vi "Control Car.vi"(8 "error in (no error)":errorcluster, 9 "Throttle":sgl, 10 "Steering":sgl, 11 "FormulaG API in":refnum<class "FormulaG API.lvclass">) -> (0 "error out":errorcluster, 3 "FormulaG API out":refnum<class "FormulaG API.lvclass">)   [LabVIEW 2020, in "FormulaG.lvlib" / "FormulaG API.lvclass"]
uses:
  FormulaG API.lvclass
  FormulaLV-Common/Car Control.ctl
  Command.ctl
  FormulaG API.lvclass/FormulaG API.ctl
  <vilib>/IlluminatedG/lv-stream/stream/Stream.lvclass/Stream.ctl
  <vilib>/IlluminatedG/lv-stream/stream/Dispatch Sniffer Data.vi
  <vilib>/IlluminatedG/lv-stream/stream/Prepared.vi
  <vilib>/IlluminatedG/lv-stream/Endpoint/Cast Sniffer Callback.vi
  <vilib>/IlluminatedG/IG WebSocket Stream/Stream-Websocket/WebsocketStream/WebsocketStream.lvclass
  C:/Program Files (x86)/National Instruments/LabVIEW 2020/vi.lib/IlluminatedG/lv-stream/stream/Stream.lvclass
  <vilib>/Utility/error.llb/Error Cluster From Error Code.vi
  <vilib>/IlluminatedG/lv-stream/stream/Stream.lvclass
  FormulaLV-Common/FormulaG-Common.lvlib
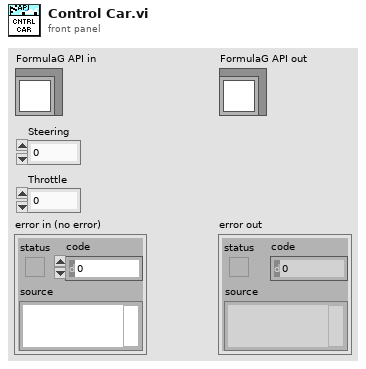
[diagram p1: front panel]
types:
  T1 = typedef "FormulaG.lvlib/FormulaG API.lvclass/Command.ctl" = enum8{"None", "Reset Car", "Request Ranges", "Control Car", "Request Info", "Set Options", "Set Camera", "Set Pause", "Request Time"}
  T2 = enum16{"big-endian, network order", "native, host order", "little-endian"}
  T3 = typedef "FormulaG-Common.lvlib/Car Control.ctl" = cluster{"Steering (-1 to 1)":sgl, "Throttle (0 to 1)":sgl}
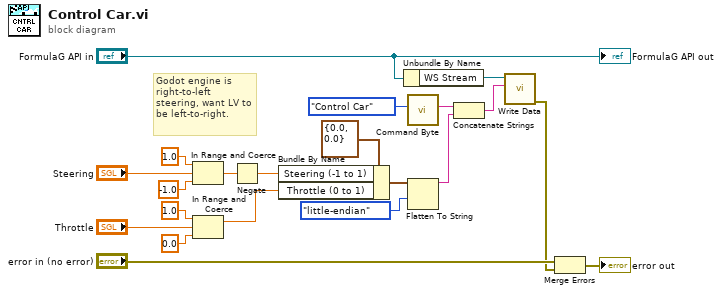
[diagram p0: block diagram]
diagram:
  # "Godot engine is right-to-left steering, want LV to be left-to-right."
  n1 = In Range and Coerce(upper limit=sgl 1.0, x="Steering", lower limit=sgl -1.0) -> (coerced(x)=w7:sgl)  [unwired: 1 out]
  n2 = In Range and Coerce(upper limit=sgl 1.0, x="Throttle", lower limit=sgl 0.0) -> (coerced(x)=w1:sgl)  [unwired: 1 out]
  n3 = Negate(x=w7) -> (-x=w18:sgl)
  n4 = Bundle By Name(cluster=T3 {"Steering (-1 to 1)"=0.0, "Throttle (0 to 1)"=0.0} ("Car Control"), "Steering (-1 to 1)"=w18, "Throttle (0 to 1)"=w1) -> (w16:T3)
  n5 = Unbundle By Name("FormulaG API in") -> ("WS Stream"=w11:refnum<class "WebsocketStream.lvclass">)
  n6 = call "Command Byte.vi"("Command"=Command."Control Car") -> ("Command Byte"=w13:string)  [unwired: 10 in]
  n7 = Flatten To String(anything=w16, byte order (0:big-endian, network order)=T2."little-endian") -> (data string=w17:string)  [unwired: 2 in, 2 out]
  n8 = Concatenate Strings(w13, w17) -> (w10:string)
  n9 = call <vilib>:"Write Data.vi"("Data"=w10, "Stream in"=w11) -> ("error out"=w8:errorcluster)  [unwired: 8 in, 1 out]
  n10 = Merge Errors("error in (no error)", w8) -> (→"error out":errorcluster)
  "FormulaG API out" <- "FormulaG API in"
